vi "zadanie_2.vi"() -> ()   [LabVIEW 2017]
panel:
  in  "?":bool
  out "Zmiana znaku r":bool
  out "Pole powierzchni kola":dbl
  in  "Promien r":dbl(slide) min=-10.0 max=10.0 scale=-10.0..10.0
  # "r"
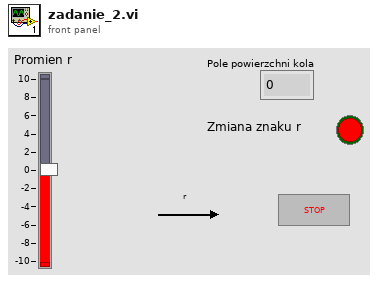
[diagram p1: front panel]
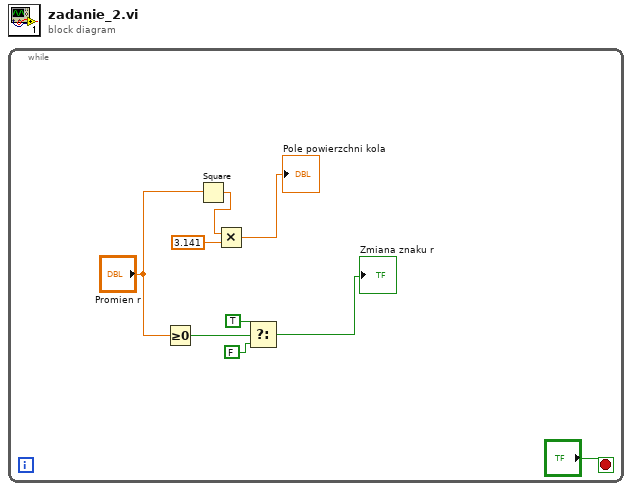
[diagram p0: block diagram]
diagram:
  n1 = while {
    stop <- "?" stop-if-true
    n2 = Greater Or Equal To 0?(x="Promien r") -> (x >= 0?=w5:bool)
    n3 = Square(x="Promien r") -> (x^2=w2:dbl)
    n4 = Multiply(x=w2, y=3.141) -> (x*y=→"Pole powierzchni kola":dbl)
    n5 = Select(t=TRUE, s=w5, f=FALSE) -> (s? t:f=→"Zmiana znaku r":bool)
  }
